vi "Get PublicEvents.vi"(8 "error in (no error)":errorcluster, 11 "SMOFacade in":refnum<class "SMOFacade.lvclass">) -> (0 "error out":errorcluster, 2 "PublicEvents":refnum<class "PublicEvents.lvclass">, 3 "SMOFacade out":refnum<class "SMOFacade.lvclass">)   [LabVIEW 2019, in "SMOFacade.lvclass"]
doc: "JKI State Machine Objects (SMO) 1.3.0.56\nJKI - JKI\nCopyright (c) 2017, JKI"
uses:
  SMOFacade.lvclass
  PublicEvents/PublicEvents.lvclass
  SMOFacade.lvclass/SMOFacade.ctl
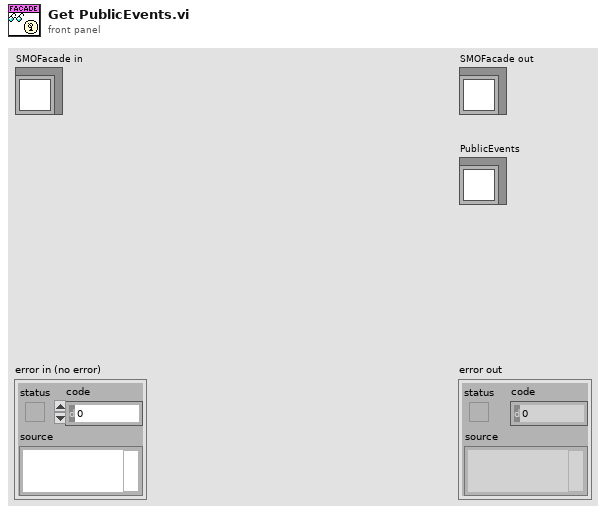
[diagram p1: front panel]
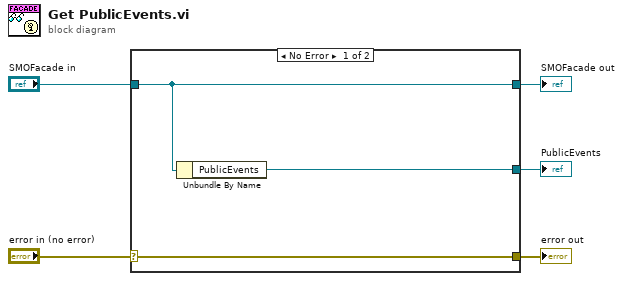
[diagram p0: block diagram]
diagram:
  n1 = case shown="No Error" "error in (no error)" {
    selector: "error in (no error)" -> [w8 w9]
    tunnel: [w8 w9] -> w4
    tunnel: [w7 w10] -> w2
    tunnel: "SMOFacade in" -> [w7 w10]
    tunnel: [w6 _] -> w1
    frame No Error {
      n2 = Unbundle By Name(w7) -> ("PublicEvents"=w6:refnum<class "PublicEvents.lvclass">)
    }
    frame Error {
    }
  }
  "error out" <- w4
  "SMOFacade out" <- w2
  "PublicEvents" <- w1
